vi "Get Selected Outputs Array.vi"(1 "UI Refs in":T1, 5 "CD Settings in":T2 {"CD Task Dependency Ref" format="%.0x"; "CD Task Dependency" format="%.0x"}, 11 "error in":errorcluster) -> (4 "Min":bool[](array[boolean]), 6 "Max":bool[](array[boolean]), 8 "SP":bool[](array[boolean]), 10 "RMS":bool[](array[boolean]), 15 "error out":errorcluster)   [LabVIEW 2017, in "Waveform-Processing-Custom-Device System Explorer.lvlib"]
doc: "This updates the arrays for the selected wavefroms, the output arrays are the Min, Max, SP, RMS, and the selected wavefrom channel names"
uses:
  Waveform-Processing-Custom-Device System Explorer.lvlib
  Shared/Custom Device Settings.ctl
  <vilib>/NI Veristand/Custom Device API/Custom Device Item Ref.ctl
  Types/UI Refs Ctl.ctl
  Types/Waveform Group Tasks.ctl
  Types/Channel Selection Array.ctl
  Types/Channel Select items.ctl
  Types/Select Buttons.ctl
  <vilib>/NI VeriStand/Custom Device API/Custom Device API.lvlib
  Shared/Waveform-Processing-Custom-Device Shared.lvlib
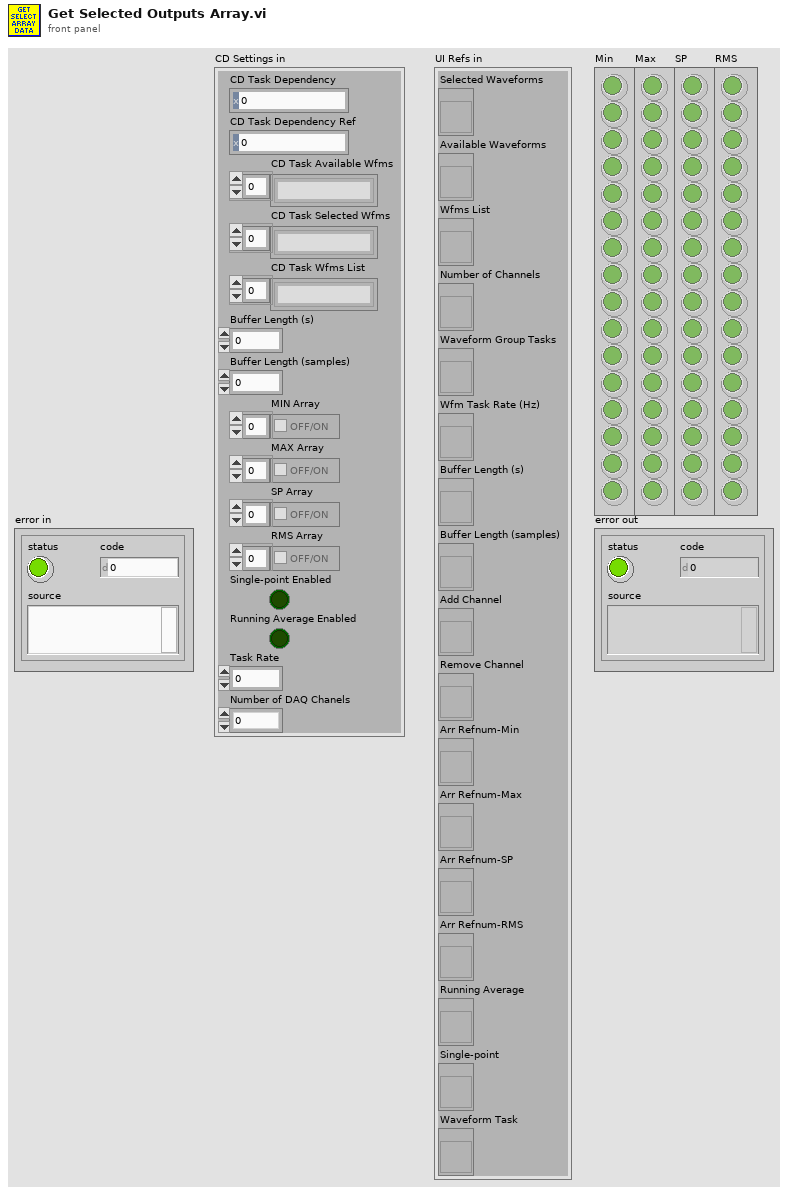
[diagram p1: front panel]
types:
  T1 = typedef "Waveform-Processing-Custom-Device Shared.lvlib/UI Refs Ctl.ctl" = cluster{"Selected Waveforms":refnum<vi>, "Available Waveforms":refnum<vi>, "Wfms List":refnum<vi>, "Number of Channels":refnum<vi>, "Waveform Group Tasks":refnum<vi>, "Wfm Task Rate (Hz)":refnum<vi>, "Buffer Length (s)":refnum<vi>, "Buffer Length (samples)":refnum<vi>, "Add Channel":refnum<vi>, "Remove Channel":refnum<vi>, "Arr Refnum-Min":refnum<vi>, "Arr Refnum-Max":refnum<vi>, "Arr Refnum-SP":refnum<vi>, "Arr Refnum-RMS":refnum<vi>, "Running Average":refnum<vi>, "Single-point":refnum<vi>, "Waveform Task":refnum<vi>}
  T2 = typedef "Waveform-Processing-Custom-Device Shared.lvlib/Custom Device Settings.ctl" = cluster{"CD Task Dependency":T3, "CD Task Dependency Ref":T3, "CD Task Available Wfms":string[], "CD Task Selected Wfms":string[], "CD Task Wfms List":string[], "Buffer Length (s)":dbl, "Buffer Length (samples)":u32, "MIN Array":bool[], "MAX Array":bool[], "SP Array":bool[], "RMS Array":bool[], "Single-point Enabled":bool, "Running Average Enabled":bool, "Task Rate":dbl, "Number of DAQ Chanels":u32}
  T3 = typedef "Custom Device API.lvlib/Custom Device Item Ref.ctl" = u64
  T4 = typedef "Waveform-Processing-Custom-Device System Explorer.lvlib/Wavefrom Task Group.ctl" = cluster{"Channel Selection Array":T5, "Buttons":T7}
  T5 = typedef "Waveform-Processing-Custom-Device System Explorer.lvlib/Channel Selection Array.ctl" = T6[]
  T6 = typedef "Waveform-Processing-Custom-Device System Explorer.lvlib/Channel Select items.ctl" = cluster{"Buttons":T7, "CH Name":string}
  T7 = typedef "Waveform-Processing-Custom-Device System Explorer.lvlib/Select Buttons.ctl" = cluster{"Min":bool, "Max":bool, "SP":bool, "RMS":bool}
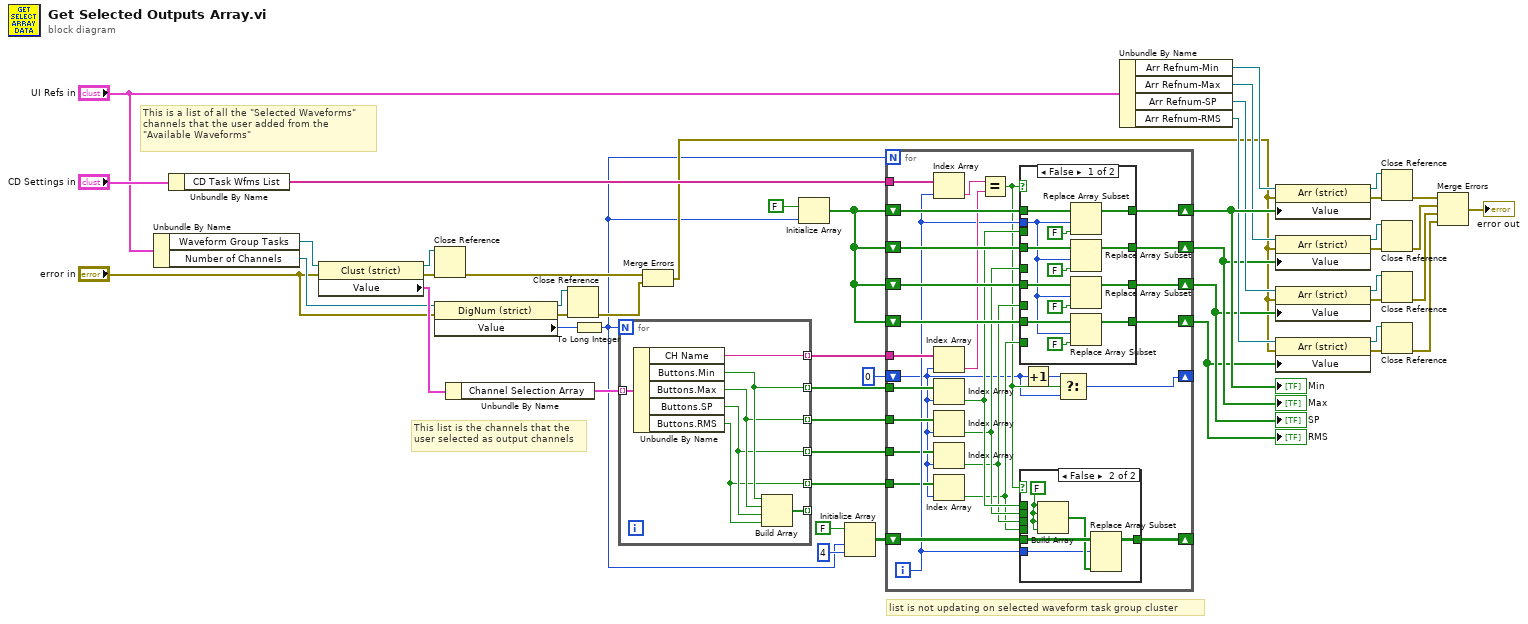
[diagram p0: block diagram]
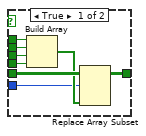
[diagram p2: hidden frame]
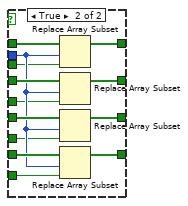
[diagram p3: hidden frame]
diagram:
  # "This list is the channels that the \nuser selected as output channels"
  # "This is a list of all the \"Selected Waveforms\" \nchannels that the user added from the \n\"Available Waveforms\""
  # "list is not updating on selected waveform task group cluster"
  n1 = Unbundle By Name("UI Refs in") -> ("Waveform Group Tasks"=w45:refnum<vi>, "Number of Channels"=w7:refnum<vi>)
  n2 = Unbundle By Name("CD Settings in") -> ("CD Task Wfms List"=w30:string[])
  n3 = property class="Clust (strict)"(reference=w45, error in="error in") -> (reference out=w47:refnum<vi>, error out=w46:errorcluster, "Value"=w48:T4)
  n4 = Close Reference(reference=w47, error in (no error)=w46) -> (error out=w9:errorcluster)
  n5 = property class="DigNum (strict)"(reference=w7, error in="error in") -> (reference out=w8:refnum<vi>, error out=w6:errorcluster, "Value"=w2:u32)
  n6 = Unbundle By Name(w48) -> ("Channel Selection Array"=w31:T5)
  n7 = Close Reference(reference=w8, error in (no error)=w6) -> (error out=w4:errorcluster)
  n8 = To Long Integer(number=w2) -> (32bit integer=w1:i32)
  n9 = for {
    N: w1 -> [_]
    tunnel: w31 -> [w56] mode=indexing
    tunnel: [w55] -> w42 mode=indexing
    tunnel: [w54] -> w41 mode=indexing
    tunnel: [w53] -> w40 mode=indexing
    tunnel: [w52] -> w39 mode=indexing
    tunnel: [w51] -> _ mode=indexing
    tunnel: [w50] -> w32 mode=indexing
    n10 = Unbundle By Name(w56) -> ("CH Name"=w50:string, "Buttons.Min"=w55:bool, "Buttons.Max"=w54:bool, "Buttons.SP"=w53:bool, "Buttons.RMS"=w52:bool)
    n11 = Build Array(w55, w54, w53, w52) -> (w51:bool[])
  }
  n12 = Merge Errors(w9, w4) -> (w5:errorcluster)
  n13 = Initialize Array(FALSE, w1) -> (w37:bool[])
  n14 = Initialize Array(FALSE, w1, 4 ("dimension size")) -> (w36:bool[][])
  n15 = for {
    N: w1 -> [_]
    tunnel: w32 -> [w71]
    tunnel: w42 -> [w67]
    tunnel: w41 -> [w64]
    tunnel: w40 -> [w61]
    tunnel: w39 -> [w59]
    shift-right: [w82] -> w26
    shift-left: w37 -> [w83]
    shift-right: [w79] -> w16
    shift-left: w37 -> [w80]
    shift-right: [w78] -> w15
    shift-left: w37 -> [w76]
    shift-right: [w77] -> w14
    shift-left: w37 -> [w75]
    tunnel: w30 -> [w74]
    shift-right: [w72] -> _
    shift-left: w36 -> [w73]
    shift-right: [w69] -> _
    shift-left: 0 ("dimension size") -> [w57]
    i -> [w63]
    n16 = Index Array(array=w74, index=w63) -> (element=w81:string)
    n17 = Index Array(array=w71, index=w57) -> (element=w70:string)
    n18 = Index Array(array=w67, index=w57) -> (element=w66:bool)
    n19 = Index Array(array=w64, index=w57) -> (element=w65:bool)
    n20 = Index Array(array=w61, index=w57) -> (element=w62:bool)
    n21 = Index Array(array=w59, index=w57) -> (element=w60:bool)
    n22 = Equal?(x=w81, y=w70) -> (x = y?=w58:bool)
    n23 = case shown="False" w58 {
      tunnel: w83 -> [w109 w122]
      tunnel: [w106 w121] -> w82
      tunnel: w63 -> [w97 w114]
      tunnel: w80 -> [w105 w120]
      tunnel: [w102 w119] -> w79
      tunnel: [w101 w118] -> w78
      tunnel: [w100 w117] -> w77
      tunnel: w76 -> [w99 w116]
      tunnel: w75 -> [w98 w115]
      tunnel: w66 -> [_ w113]
      tunnel: w65 -> [_ w112]
      tunnel: w62 -> [_ w111]
      tunnel: w60 -> [_ w110]
      frame False {
        n24 = Replace Array Subset(array=w109, new element=FALSE ("new element/subarray"), index=w97) -> (w106:bool[])
        n25 = Replace Array Subset(array=w105, new element=FALSE ("new element/subarray"), index=w97) -> (w102:bool[])
        n26 = Replace Array Subset(array=w99, new element=FALSE ("new element/subarray"), index=w97) -> (w101:bool[])
        n27 = Replace Array Subset(array=w98, new element=FALSE ("new element/subarray"), index=w97) -> (w100:bool[])
      }
      frame True {
        n28 = Replace Array Subset(array=w122, new element=w113, index=w114) -> (w121:bool[])
        n29 = Replace Array Subset(array=w120, new element=w112, index=w114) -> (w119:bool[])
        n30 = Replace Array Subset(array=w116, new element=w111, index=w114) -> (w118:bool[])
        n31 = Replace Array Subset(array=w115, new element=w110, index=w114) -> (w117:bool[])
      }
    }
    n32 = case shown="False" w58 {
      tunnel: w73 -> [w91 w96]
      tunnel: [w90 w95] -> w72
      tunnel: w66 -> [w88 _]
      tunnel: w65 -> [w87 _]
      tunnel: w63 -> [w86 w93]
      tunnel: w62 -> [w85 _]
      tunnel: w60 -> [w84 _]
      frame True {
        n33 = Build Array(w88, w87, w85, w84) -> (w89:bool[])
        n34 = Replace Array Subset(array=w91, new element=w89, index (row)=w86) -> (w90:bool[][])  [unwired: 1 in]
      }
      frame False {
        w92 = FALSE
        n35 = Build Array(w92, w92, w92, w92) -> (w94:bool[])
        n36 = Replace Array Subset(array=w96, new element=w94, index (row)=w93) -> (w95:bool[][])  [unwired: 1 in]
      }
    }
    n37 = Increment(x=w57) -> (x+1=w68:i32)
    n38 = Select(t=w68, s=w58, f=w57) -> (s? t:f=w69:i32)
  }
  "Min" <- w26
  "Max" <- w16
  "SP" <- w15
  "RMS" <- w14
  n39 = Unbundle By Name("UI Refs in") -> ("Arr Refnum-Min"=w27:refnum<vi>, "Arr Refnum-Max"=w19:refnum<vi>, "Arr Refnum-SP"=w18:refnum<vi>, "Arr Refnum-RMS"=w17:refnum<vi>)
  n40 = property class="Arr (strict)"(reference=w27, error in=w5, "Value"=w26) -> (reference out=w44:refnum<vi>, error out=w43:errorcluster)
  n41 = property class="Arr (strict)"(reference=w19, error in=w5, "Value"=w16) -> (reference out=w24:refnum<vi>, error out=w25:errorcluster)
  n42 = property class="Arr (strict)"(reference=w18, error in=w5, "Value"=w15) -> (reference out=w23:refnum<vi>, error out=w22:errorcluster)
  n43 = property class="Arr (strict)"(reference=w17, error in=w5, "Value"=w14) -> (reference out=w20:refnum<vi>, error out=w21:errorcluster)
  n44 = Close Reference(reference=w44, error in (no error)=w43) -> (error out=w29:errorcluster)
  n45 = Close Reference(reference=w24, error in (no error)=w25) -> (error out=w12:errorcluster)
  n46 = Close Reference(reference=w23, error in (no error)=w22) -> (error out=w11:errorcluster)
  n47 = Close Reference(reference=w20, error in (no error)=w21) -> (error out=w10:errorcluster)
  n48 = Merge Errors(w29, w12, w11, w10) -> (→"error out":errorcluster)
